vi "DeviceWrite.vi"(1 "error in":errorcluster, 2 "nbytes":i32, 3 "buffer":u8[](array[numeric]), 4 "handle":i32) -> (0 "FTC_Status":u32)   [LabVIEW 2010]
uses:
  WINNT/system32/FTCSPI.dll
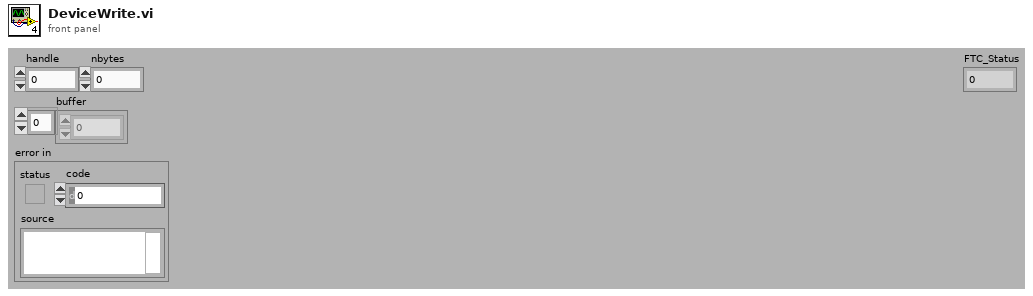
[diagram p1: front panel]
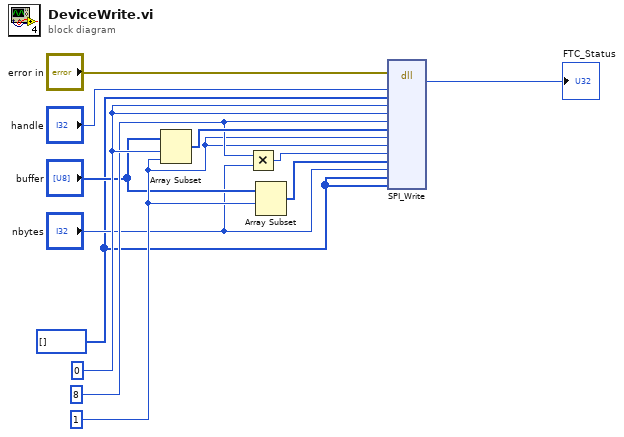
[diagram p0: block diagram]
diagram:
  w6 = 1 ("length")
  w7 = u32 8 ("NumControlBitsToWrite")
  w10 = u32 0 ("ClockOutControlBitsMSBFirst")
  w2 = u8[] [] ("buffer 2")
  n1 = Array Subset(array="buffer", index=w10, length=w6) -> (w9:u8[])
  n2 = Multiply(x=w7, y="nbytes") -> (x*y=w8:u32)
  n3 = Array Subset(array="buffer", index=w6) -> (w4:u8[])  [unwired: 1 in]
  n4 = dll-call lib="C:/Users/WINNT/system32/FTCSPI.dll" fn="SPI_Write"(error in="error in", "Handle"="handle", w2, "ClockOutControlBitsMSBFirst"=w10, "ClockOutControlBitsPosEdge"=w10, "NumControlBitsToWrite"=w7, "WriteControlBuffer"=w9, "NumControlBytesToWrite"=w6, "WriteDataBits"=w6, "NumDataBitsToWrite"=w8, "WriteDataBuffer"=w4, "NumDataBytesToWrite"="nbytes", w2, w2) -> ("FTC_Status"=→"FTC_Status":u32)  [unwired: 15 in, 2 out]
